vi "Tag Transactions.vi"(10 "Transactions In":T1[](array[typedef]), 11 "Force Tag":string) -> (2 "Transactions Out":T1[](array[typedef]))   [LabVIEW 2009]
uses:
  Dataset Transaction Id.ctl
  Dataset Source.ctl
  Dataset Type.ctl
  Apps/Yes No Button.ctl
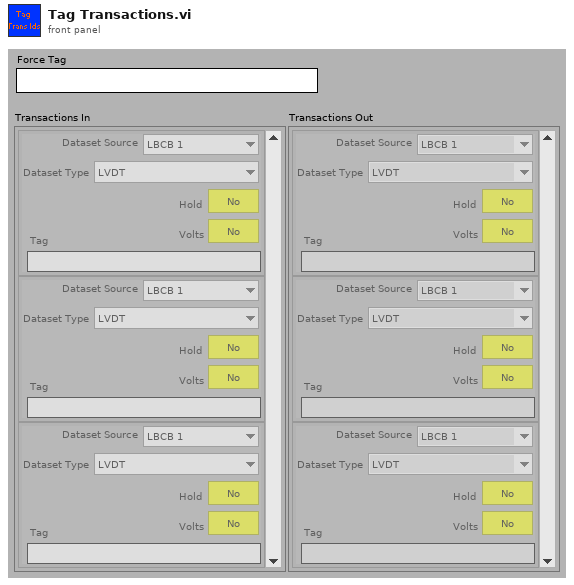
[diagram p1: front panel]
types:
  T1 = typedef "Dataset Transaction Id.ctl" = cluster{"Dataset Source":T2, "Dataset Type":T3, "Hold":T4, "Volts":T4, "Tag":string}
  T2 = typedef "Dataset Source.ctl" = enum16{"LBCB 1", "LBCB 2", "Combined", "External Sensors"}
  T3 = typedef "Dataset Type.ctl" = enum16{"LVDT", "Load Cell", "Actuator Command", "Servo Error", "Displacement Command", "Displacement", "Force"}
  T4 = typedef "Yes No Button.ctl" = bool
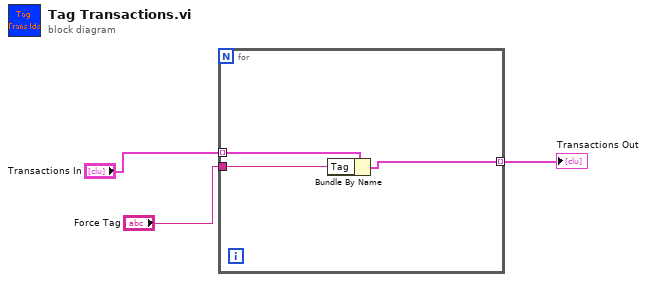
[diagram p0: block diagram]
diagram:
  n1 = for {
    tunnel: "Transactions In" -> [w6] mode=indexing
    tunnel: "Force Tag" -> [w5]
    tunnel: [w4] -> w1 mode=indexing
    n2 = Bundle By Name(cluster=w6, "Tag"=w5) -> (w4:T1)
  }
  "Transactions Out" <- w1
